vi "Read Decoration Index.vi"(3 "DecFrame_FP":refnum<class "DecFrame_FP.lvclass">) -> (1 "Decoration Index":i32)   [LabVIEW 2023, in "DecFrame_FP.lvclass"]
uses:
  DecFrame_FP.lvclass
  DecFrame_FP.lvclass/DecFrame_FP.ctl
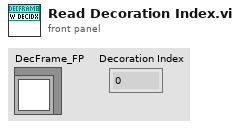
[diagram p1: front panel]
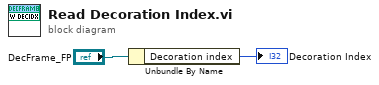
[diagram p0: block diagram]
diagram:
  n1 = Unbundle By Name("DecFrame_FP") -> ("Decoration index"=→"Decoration Index":i32)
